vi "VISP PNG Read.vi"(8 "error in (no error)":errorcluster, 11 "Image Path (*.png)":path) -> (0 "error out":errorcluster, 2 "Chunks":T1[](array[typedef]) {"CRC" format="%08x"}, 3 "dup Image Path":path)   [LabVIEW 2019, in "VI Snippet.lvlib"]
doc: "Returns the PNG image chunks from the <b>Image Path (*.png)</b>.\n\n<b>Errors:</b>\n1059: \"Unsupported file type\" if <b>Image Path (*.png)</b> is not a valid PNG file.\n\nCreated by: Ryan Pacini"
uses:
  VI Snippet.lvlib
  VISP PNG Chunk.ctl
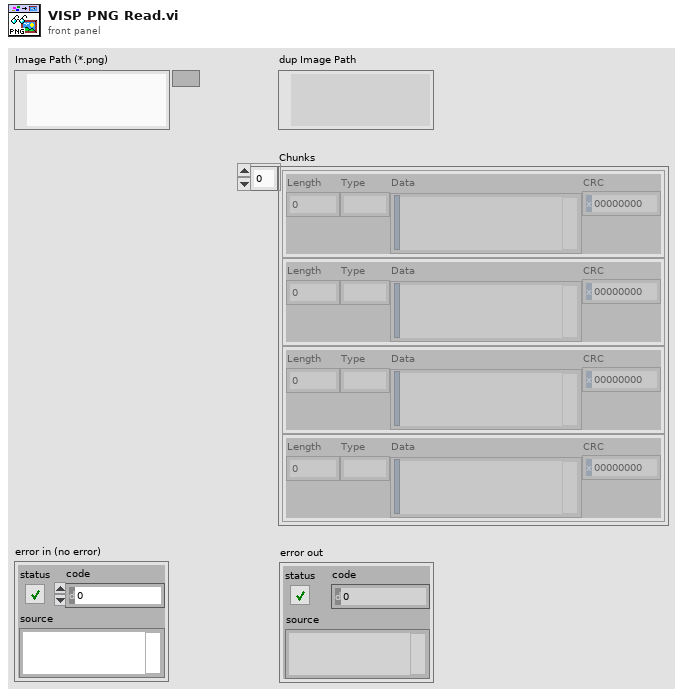
[diagram p1: front panel]
types:
  T1 = typedef "VI Snippet.lvlib/VISP PNG Chunk.ctl" = cluster{"Length":i32, "Type":string, "Data":string, "CRC":u32}
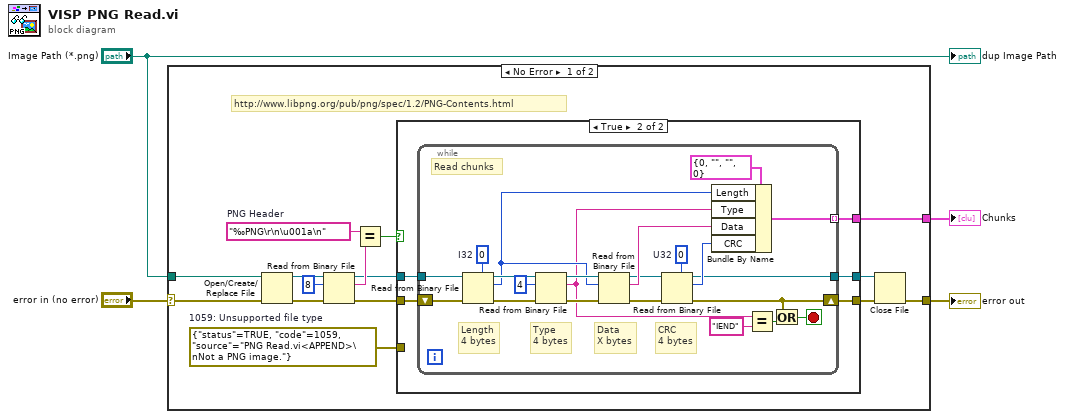
[diagram p0: block diagram]
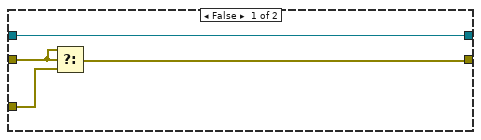
[diagram p2: hidden frame]
diagram:
  n1 = case shown="No Error" "error in (no error)" {
    selector: "error in (no error)" -> [w19 w51]
    tunnel: "Image Path (*.png)" -> [w18 _]
    tunnel: [w12 _] -> w2
    tunnel: [w10 w51] -> w3
    frame No Error {
      w5 = errorcluster {"status"=TRUE, "code"=1059, "source"="PNG Read.vi<APPEND>\nNot a PNG image."}  # 1059: Unsupported file type
      w6 = "‰PNG\r\n\u001a\n"  # PNG Header
      # "http://www.libpng.org/pub/png/spec/1.2/PNG-Contents.html"
      n2 = Open/Create/Replace File(file path (use dialog)=w18, error in=w19) -> (refnum out=w17:refnum<file>, error out=w16:errorcluster)  [unwired: 4 in, 1 out]
      n3 = Read from Binary File(8:w16, 10:8 ("count (1)"), 11:w17) -> (0:w14:errorcluster, 2:w15:string, 3:w13:refnum<file>)  [unwired: 3 in, 1 out]
      n4 = Equal?(x=w6, y=w15) -> (x = y?=w8:bool)
      n5 = case shown="True" w8 {
        tunnel: w14 -> [w22 w28]
        tunnel: w13 -> [w23 w27]
        tunnel: [_ w26] -> w12
        tunnel: [w20 w25] -> w11
        tunnel: [w23 w24] -> w9
        tunnel: w5 -> [w21 _]
        frame False {
          n6 = Select(t=w22, s=w22, f=w21) -> (s? t:f=w20:errorcluster)
        }
        frame True {
          n7 = while {
            tunnel: w27 -> [w49]
            tunnel: [w47] -> w26 mode=indexing
            shift-right: [w35] -> w25
            shift-left: w28 -> [w50]
            tunnel: [w31] -> w24
            stop <- w32 stop-if-true
            w37 = u32 0  # U32
            w48 = 0  # I32
            # "Read chunks"
            # "CRC\n4 bytes"
            # "Data\nX bytes"
            # "Type\n4 bytes"
            # "Length\n4 bytes"
            n8 = Read from Binary File(5:w48, 8:w50, 11:w49) -> (0:w46:errorcluster, 2:w41:i32, 3:w45:refnum<file>)  [unwired: 3 in, 1 out]
            n9 = Read from Binary File(8:w46, 10:4 ("count (1)"), 11:w45) -> (0:w43:errorcluster, 2:w34:string, 3:w42:refnum<file>)  [unwired: 3 in, 1 out]
            n10 = Read from Binary File(8:w43, 10:w41, 11:w42) -> (0:w39:errorcluster, 2:w40:string, 3:w38:refnum<file>)  [unwired: 3 in, 1 out]
            n11 = Read from Binary File(5:w37, 8:w39, 11:w38) -> (0:w35:errorcluster, 2:w36:u32, 3:w31:refnum<file>)  [unwired: 3 in, 1 out]
            n12 = Bundle By Name(cluster=T1 {"Length"=0, "Type"="", "Data"="", "CRC"=0} ("Chunk"), "Length"=w41, "Type"=w34, "Data"=w40, "CRC"=w36) -> (w47:T1)
            n13 = Equal?(x=w34, y="IEND") -> (x = y?=w33:bool)
            n14 = Or(x=w35, y=w33) -> (x .or. y?=w32:bool)
          }
        }
      }
      n15 = Close File(refnum=w9, error in=w11) -> (error out=w10:errorcluster)  [unwired: 1 out]
    }
    frame Error {
    }
  }
  "error out" <- w3
  "Chunks" <- w2
  "dup Image Path" <- "Image Path (*.png)"
